vi "biref2.vi"() -> ()   [LabVIEW 2025]
doc: "Author: Scott Hannahs <sth@magnet.fsu.edu>\n\nThis software is licensed for use under the “MIT License\"\nCopyright (c) 2025 Scott Hannahs, sth@sth@magnet.sthnet.net\n\nPermission is hereby granted, free of charge, to any person obtaining a copy of this software and associated documentation files (the \"Software\"), to deal in the Software without restriction, including without limitation the rights to use, copy, modify, merge, publish, distribute, sublicense, and/or sell copies of the Software, and to permit persons to whom the Software is furnished to do so, subject to the following conditions: The above copyright notice and this permission notice shall be included in all copies or substantial portions of the Software.\n\nTHE SOFTWARE IS PROVIDED \"AS IS\", WITHOUT WARRANTY OF ANY KIND, EXPRESS OR IMPLIED, INCLUDING BUT NOT LIMITED TO THE WARRANTIES OF MERCHANTABILITY, FITNESS FOR A PARTICULAR PURPOSE AND NONINFRINGEMENT. IN NO EVENT SHALL THE AUTHORS OR COPYRIGHT HOLDERS BE LIABLE FOR ANY CLAIM, DAMAGES OR OTHER LIABILITY, WHETHER IN AN ACTION OF CONTRACT, TORT OR OTHERWISE, ARISING FROM, OUT OF OR IN CONNECTION WITH THE SOFTWARE OR THE USE OR OTHER DEALINGS IN THE SOFTWARE."
panel:
  in  "Case Constant\n(See Context Help)":bool
  in  "folder name":string
  in  "field increment":dbl
  out "Current field":dbl
  in  "Initial field T":dbl=0.08
  in  "No  Steps":i16
  out "outputdc 2":dbl[](array[numeric]) format="%.2f"
  in  "GPIB address dc meter 2":string="2"
  in  "GPIB address dc meter":string="5"
  in  "GPIB  address  lockin":string="3"
  in  "GPIB address magnet":string="1"
  in  "GPIB address Temp controller":string="12"
  in  "Wait (second)":sgl
  in  "No of Temp Steps":i16
  out "outputtemp":dbl[](array[numeric]) format="%.2f"
  out "outputdc":dbl[](array[numeric]) format="%.2f"
  out "outputlockin 2":dbl[](array[numeric]) format="%.2f"
  out "outputlockin 1":dbl[](array[numeric]) format="%.2f"
  out "field":dbl[](array[numeric]) format="%.2f"
  out "Current Temp":dbl format="%.3f"
  in  "Increasing \nTemp step":bool=TRUE
  in  "Initial Temp C":dbl format="%.3f"
  # "Help:\n1. write the folder name to save the files.The file name will \nbe the temperature in the given folder.\n2.Write the GPIB address of all the instruments before running\nthe program.\n3. Give the initial temperature and the temperature interval \nand the total number of steps.\n4.Check whether you want to increase the temperature or\ndecrease.\n5.Write the time to be waited to let the tempetature controller\nequilibrate.\n6.Once the speps 1 through 5 is done run the experiment."
  # "Decreasing\nTemp Step"
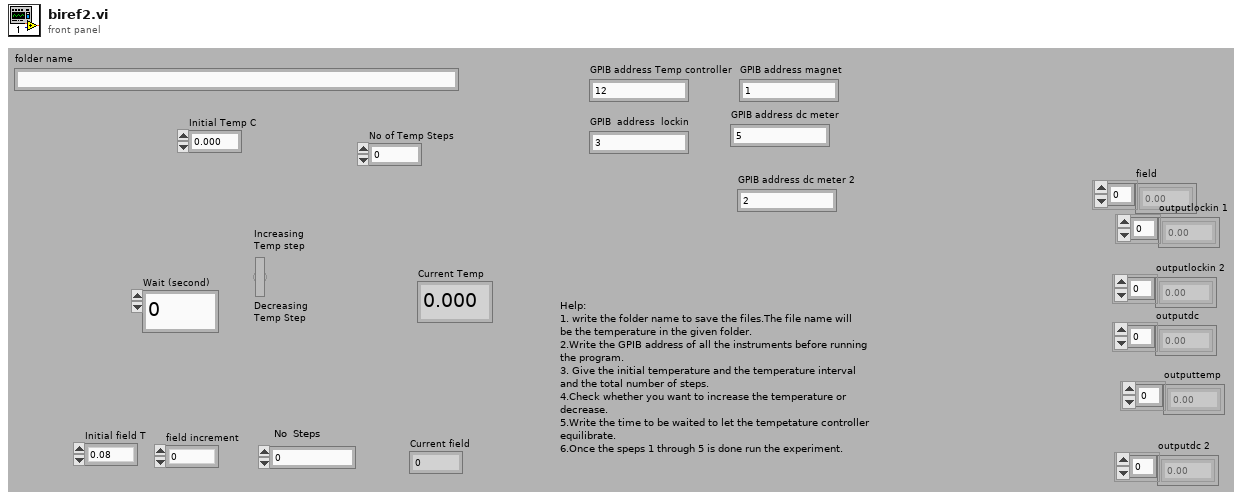
[diagram p1: front panel]
types:
  T1 = enum16{"--Quit--", "Read-Status", "Read-Cell", "Read-Field[T]", "Read-Setpoint[T]"}
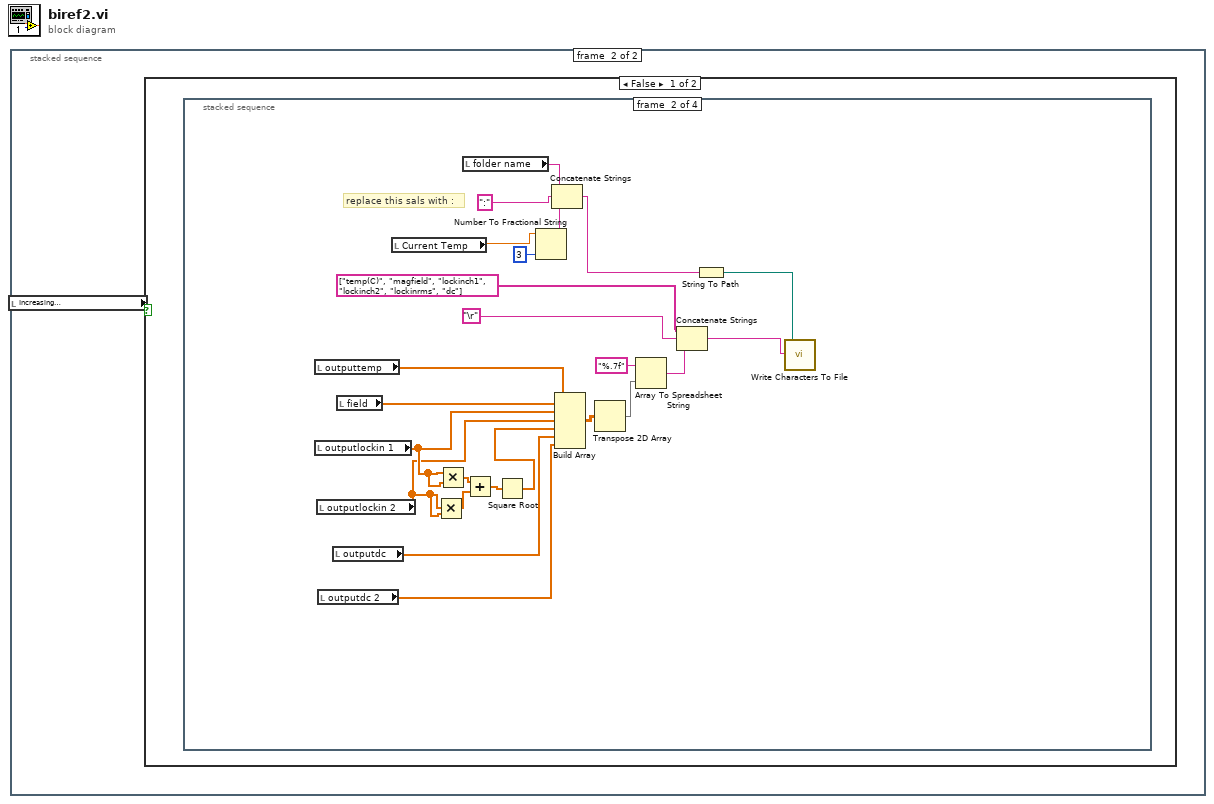
[diagram p0: block diagram]
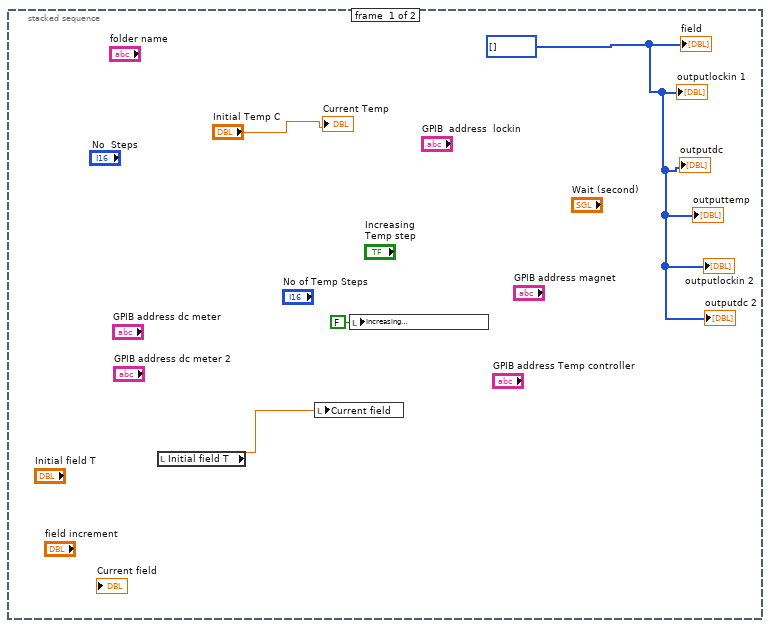
[diagram p2: hidden frame]
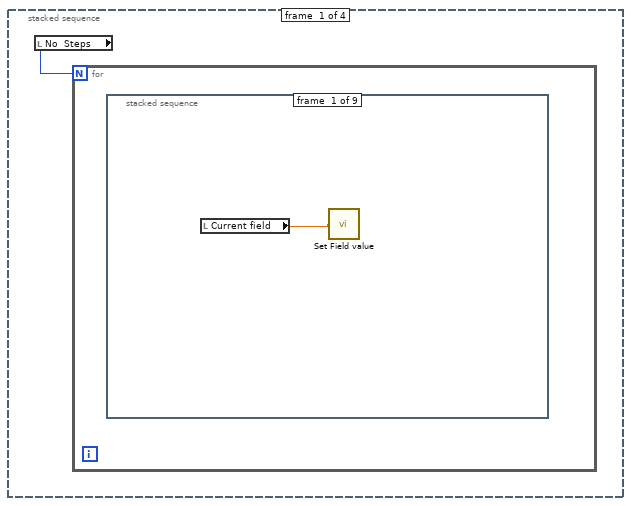
[diagram p3: hidden frame]
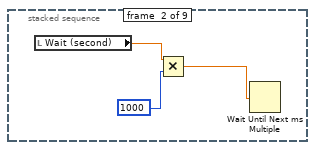
[diagram p4: hidden frame]
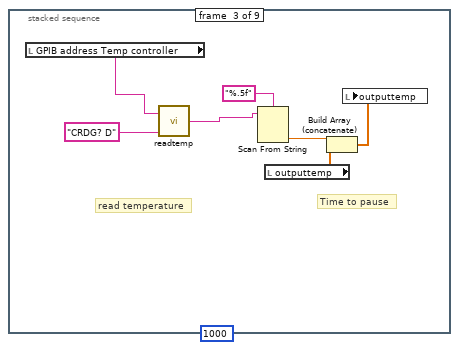
[diagram p5: hidden frame]
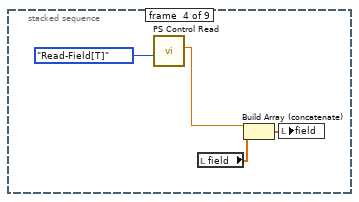
[diagram p6: hidden frame]
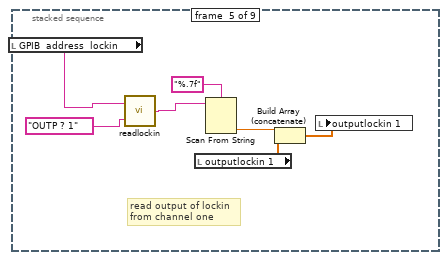
[diagram p7: hidden frame]
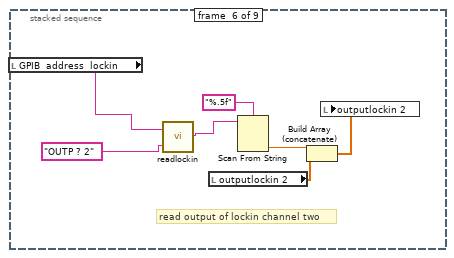
[diagram p8: hidden frame]
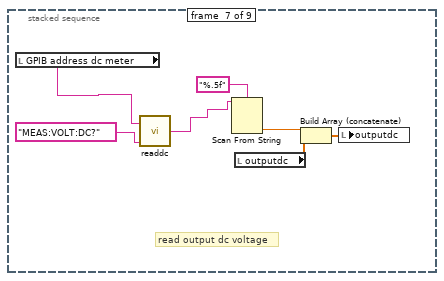
[diagram p9: hidden frame]
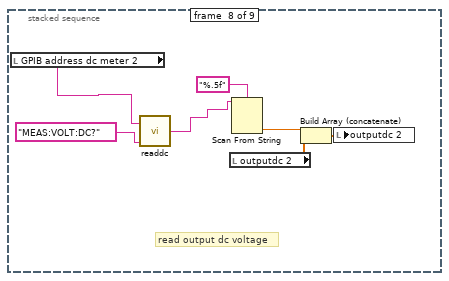
[diagram p10: hidden frame]
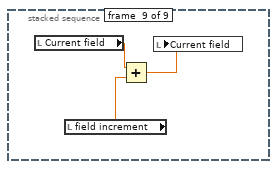
[diagram p11: hidden frame]
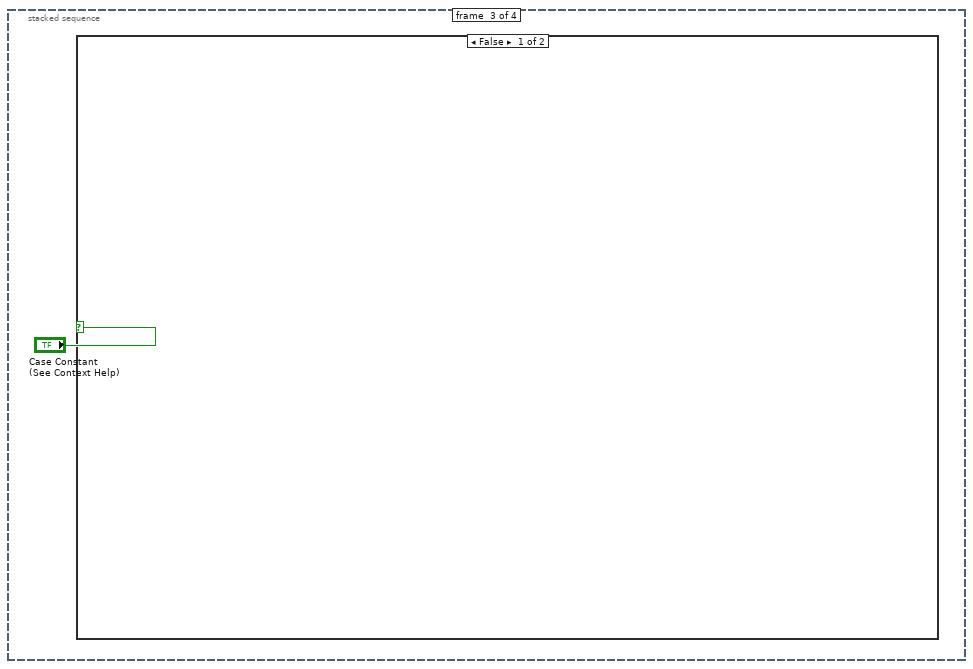
[diagram p12: hidden frame]
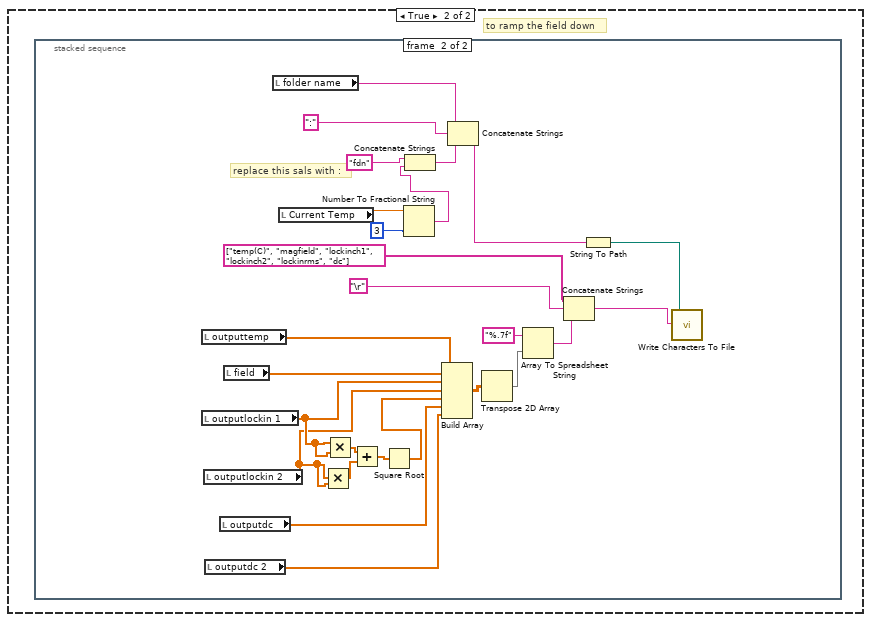
[diagram p13: hidden frame]
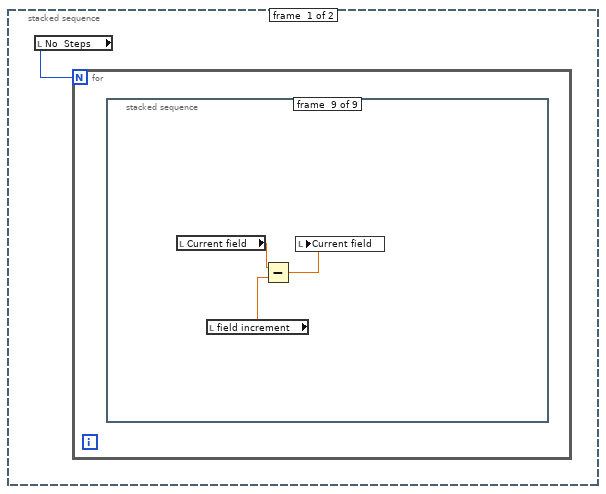
[diagram p14: hidden frame]
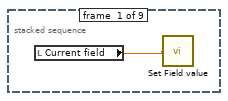
[diagram p15: hidden frame]
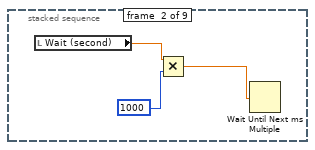
[diagram p16: hidden frame]
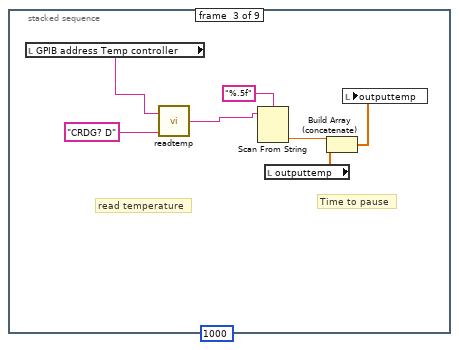
[diagram p17: hidden frame]
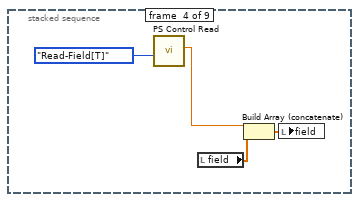
[diagram p18: hidden frame]
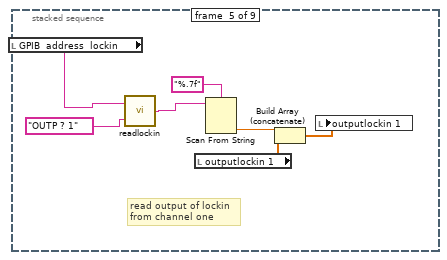
[diagram p19: hidden frame]
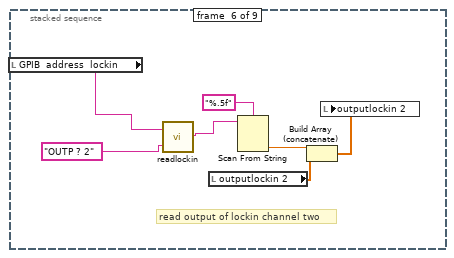
[diagram p20: hidden frame]
diagram:
  n1 = stacked-sequence {
    frame #0 {
      w3 = i32[] [] ("field")
      n2 = local read "Initial field T"() -> (w1:dbl)
      n3 = local write "Current field"(w1) -> ()
      n4 = local write "Increasing \nTemp step"(FALSE ("Increasing \nTemp step")) -> ()
      "Current Temp" <- "Initial Temp C"
      "field" <- w3
      "outputlockin 1" <- w3
      "outputdc" <- w3
      "outputtemp" <- w3
      "outputlockin 2" <- w3
      "outputdc 2" <- w3
    }
    frame #1 {
      n5 = local read "Increasing \nTemp step"() -> (w5:bool)
      n6 = case shown="False" w5 {
        frame False {
          n7 = stacked-sequence {
            frame #0 {
              n8 = local read "No  Steps"() -> (w6:i16)
              n9 = for {
                N: w6 -> [_]
                n10 = stacked-sequence {
                  frame #0 {
                    n11 = local read "Current field"() -> (w7:dbl)
                    n12 = call "Set Field value.vi"("Field"=w7) -> ()
                  }
                  frame #1 {
                    n13 = local read "Wait (second)"() -> (w10:sgl)
                    n14 = Multiply(x=w10, y=u32 1000 ("millisecond multiple")) -> (x*y=w8:sgl)
                    n15 = Wait Until Next ms Multiple(millisecond multiple=w8) -> ()  [unwired: 1 out]
                  }
                  frame #2 {
                    (unwired) u32 1000 ("millisecond multiple")
                    # "Time to pause"
                    # "read temperature"
                    n16 = local read "GPIB address Temp controller"() -> (w11:string)
                    n17 = call "readtemp.vi"("Characters to Write"="CRDG? D", "GPIB\nAddress"=w11) -> ("Characters Read"=w12:string)
                    n18 = Scan From String(format string="%.5f", input string=w12) -> (output 1=w14:dbl)  [unwired: 3 in, 3 out]
                    n19 = local read "outputtemp"() -> (w17:dbl[])
                    n20 = Build Array (concatenate)(w14, w17) -> (w16:dbl[])
                    n21 = local write "outputtemp"(w16) -> ()
                  }
                  frame #3 {
                    n22 = call "PS Control Read.vi"("Read State"=T1."Read-Field[T]") -> ("Current Field"=w18:dbl)  [unwired: 3 in, 4 out]
                    n23 = local read "field"() -> (w20:dbl[])
                    n24 = Build Array (concatenate)(w18, w20) -> (w19:dbl[])
                    n25 = local write "field"(w19) -> ()
                  }
                  frame #4 {
                    # "read output of lockin\nfrom channel one"
                    n26 = local read "GPIB  address  lockin"() -> (w22:string)
                    n27 = call "readlockin.vi"("Characters to Write"="OUTP ? 1", "GPIB\nAddress"=w22) -> ("Characters Read"=w23:string)
                    n28 = local read "outputlockin 1"() -> (w27:dbl[])
                    n29 = Scan From String(format string="%.7f", input string=w23) -> (output 1=w24:dbl)  [unwired: 3 in, 3 out]
                    n30 = Build Array (concatenate)(w24, w27) -> (w26:dbl[])
                    n31 = local write "outputlockin 1"(w26) -> ()
                  }
                  frame #5 {
                    # "read output of lockin channel two"
                    n32 = local read "GPIB  address  lockin"() -> (w29:string)
                    n33 = call "readlockin.vi"("Characters to Write"="OUTP ? 2", "GPIB\nAddress"=w29) -> ("Characters Read"=w30:string)
                    n34 = local read "outputlockin 2"() -> (w34:dbl[])
                    n35 = Scan From String(format string="%.5f", input string=w30) -> (output 1=w32:dbl)  [unwired: 3 in, 3 out]
                    n36 = Build Array (concatenate)(w32, w34) -> (w33:dbl[])
                    n37 = local write "outputlockin 2"(w33) -> ()
                  }
                  frame #6 {
                    # "read output dc voltage"
                    n38 = local read "GPIB address dc meter"() -> (w36:string)
                    n39 = call "readdc.vi"("Characters to Write"="MEAS:VOLT:DC?", "GPIB\nAddress"=w36) -> ("Characters Read"=w37:string)
                    n40 = Scan From String(format string="%.5f", input string=w37) -> (output 1=w39:dbl)  [unwired: 3 in, 3 out]
                    n41 = local read "outputdc"() -> (w42:dbl[])
                    n42 = Build Array (concatenate)(w39, w42) -> (w41:dbl[])
                    n43 = local write "outputdc"(w41) -> ()
                  }
                  frame #7 {
                    # "read output dc voltage"
                    n44 = local read "GPIB address dc meter 2"() -> (w43:string)
                    n45 = call "readdc.vi"("Characters to Write"="MEAS:VOLT:DC?", "GPIB\nAddress"=w43) -> ("Characters Read"=w44:string)
                    n46 = local read "outputdc 2"() -> (w49:dbl[])
                    n47 = Scan From String(format string="%.5f", input string=w44) -> (output 1=w46:dbl)  [unwired: 3 in, 3 out]
                    n48 = Build Array (concatenate)(w46, w49) -> (w48:dbl[])
                    n49 = local write "outputdc 2"(w48) -> ()
                  }
                  frame #8 {
                    n50 = local read "Current field"() -> (w52:dbl)
                    n51 = local read "field increment"() -> (w51:dbl)
                    n52 = Add(x=w52, y=w51) -> (x+y=w50:dbl)
                    n53 = local write "Current field"(w50) -> ()
                  }
                }
              }
            }
            frame #1 {
              # "replace this sals with :"
              n54 = local read "outputtemp"() -> (w71:dbl[])
              n55 = local read "outputlockin 1"() -> (w69:dbl[])
              n56 = local read "outputlockin 2"() -> (w68:dbl[])
              n57 = local read "outputdc 2"() -> (w54:dbl[])
              n58 = local read "outputdc"() -> (w63:dbl[])
              n59 = local read "field"() -> (w70:dbl[])
              n60 = local read "Current Temp"() -> (w73:dbl)
              n61 = Multiply(x=w68, y=w68) -> (x*y=w66:dbl[])
              n62 = Multiply(x=w69, y=w69) -> (x*y=w67:dbl[])
              n63 = local read "folder name"() -> (w53:string)
              n64 = Add(x=w67, y=w66) -> (x+y=w65:dbl[])
              n65 = Square Root(x=w65) -> (sqrt(x)=w64:dbl[])
              n66 = Number To Fractional String(number=w73, precision (6)=i16 3) -> (F-format string=w72:string)  [unwired: 2 in]
              n67 = Concatenate Strings(w53, ":", w72) -> (w75:string)
              n68 = Build Array(w71, w70, w69, w68, w64, w63, w54) -> (w62:dbl[][])
              n69 = Transpose 2D Array(2D array=w62) -> (transposed array=w60:dbl[][])
              n70 = Array To Spreadsheet String(array=w60, 3:"%.7f" ("format string")) -> (spreadsheet string=w57:string)  [unwired: 1 in]
              n71 = Concatenate Strings(string[] ["temp(C)", "magfield", "lockinch1", "lockinch2", "lockinrms", "dc"], "\r", w57) -> (w56:string)
              n72 = String To Path(string=w75) -> (path=w74:path)
              n73 = call <vilib>:"Write Characters To File.vi"("character string"=w56, "file path (dialog if empty)"=w74) -> ()  [unwired: 3 in, 1 out]
            }
            frame #2 {
              n74 = case shown="False" "Case Constant\n(See Context Help)" {
                frame False {
                }
                frame True {
                  # "to ramp the field down"
                  n75 = stacked-sequence {
                    frame #0 {
                      n76 = local read "No  Steps"() -> (w78:i16)
                      n77 = for {
                        N: w78 -> [_]
                        n78 = stacked-sequence {
                          frame #0 {
                            n79 = local read "Current field"() -> (w79:dbl)
                            n80 = call "Set Field value.vi"("Field"=w79) -> ()
                          }
                          frame #1 {
                            n81 = local read "Wait (second)"() -> (w82:sgl)
                            n82 = Multiply(x=w82, y=u32 1000 ("millisecond multiple")) -> (x*y=w80:sgl)
                            n83 = Wait Until Next ms Multiple(millisecond multiple=w80) -> ()  [unwired: 1 out]
                          }
                          frame #2 {
                            (unwired) u32 1000 ("millisecond multiple")
                            # "Time to pause"
                            # "read temperature"
                            n84 = local read "GPIB address Temp controller"() -> (w83:string)
                            n85 = call "readtemp.vi"("Characters to Write"="CRDG? D", "GPIB\nAddress"=w83) -> ("Characters Read"=w84:string)
                            n86 = Scan From String(format string="%.5f", input string=w84) -> (output 1=w86:dbl)  [unwired: 3 in, 3 out]
                            n87 = local read "outputtemp"() -> (w89:dbl[])
                            n88 = Build Array (concatenate)(w86, w89) -> (w88:dbl[])
                            n89 = local write "outputtemp"(w88) -> ()
                          }
                          frame #3 {
                            n90 = call "PS Control Read.vi"("Read State"=T1."Read-Field[T]") -> ("Current Field"=w90:dbl)  [unwired: 3 in, 4 out]
                            n91 = local read "field"() -> (w92:dbl[])
                            n92 = Build Array (concatenate)(w90, w92) -> (w91:dbl[])
                            n93 = local write "field"(w91) -> ()
                          }
                          frame #4 {
                            # "read output of lockin\nfrom channel one"
                            n94 = local read "GPIB  address  lockin"() -> (w94:string)
                            n95 = call "readlockin.vi"("Characters to Write"="OUTP ? 1", "GPIB\nAddress"=w94) -> ("Characters Read"=w95:string)
                            n96 = local read "outputlockin 1"() -> (w99:dbl[])
                            n97 = Scan From String(format string="%.7f", input string=w95) -> (output 1=w96:dbl)  [unwired: 3 in, 3 out]
                            n98 = Build Array (concatenate)(w96, w99) -> (w98:dbl[])
                            n99 = local write "outputlockin 1"(w98) -> ()
                          }
                          frame #5 {
                            # "read output of lockin channel two"
                            n100 = local read "GPIB  address  lockin"() -> (w101:string)
                            n101 = call "readlockin.vi"("Characters to Write"="OUTP ? 2", "GPIB\nAddress"=w101) -> ("Characters Read"=w102:string)
                            n102 = local read "outputlockin 2"() -> (w106:dbl[])
                            n103 = Scan From String(format string="%.5f", input string=w102) -> (output 1=w104:dbl)  [unwired: 3 in, 3 out]
                            n104 = Build Array (concatenate)(w104, w106) -> (w105:dbl[])
                            n105 = local write "outputlockin 2"(w105) -> ()
                          }
                          frame #6 {
                            # "read output dc voltage"
                            n106 = local read "GPIB address dc meter"() -> (w108:string)
                            n107 = call "readdc.vi"("Characters to Write"="MEAS:VOLT:DC?", "GPIB\nAddress"=w108) -> ("Characters Read"=w109:string)
                            n108 = Scan From String(format string="%.5f", input string=w109) -> (output 1=w111:dbl)  [unwired: 3 in, 3 out]
                            n109 = local read "outputdc"() -> (w114:dbl[])
                            n110 = Build Array (concatenate)(w111, w114) -> (w113:dbl[])
                            n111 = local write "outputdc"(w113) -> ()
                          }
                          frame #7 {
                            # "read output dc voltage"
                            n112 = local read "GPIB address dc meter 2"() -> (w115:string)
                            n113 = call "readdc.vi"("Characters to Write"="MEAS:VOLT:DC?", "GPIB\nAddress"=w115) -> ("Characters Read"=w116:string)
                            n114 = local read "outputdc 2"() -> (w121:dbl[])
                            n115 = Scan From String(format string="%.5f", input string=w116) -> (output 1=w118:dbl)  [unwired: 3 in, 3 out]
                            n116 = Build Array (concatenate)(w118, w121) -> (w120:dbl[])
                            n117 = local write "outputdc 2"(w120) -> ()
                          }
                          frame #8 {
                            n118 = local read "Current field"() -> (w124:dbl)
                            n119 = local read "field increment"() -> (w123:dbl)
                            n120 = Subtract(x=w124, y=w123) -> (x-y=w122:dbl)
                            n121 = local write "Current field"(w122) -> ()
                          }
                        }
                      }
                    }
                    frame #1 {
                      # "replace this sals with :"
                      n122 = local read "outputtemp"() -> (w146:dbl[])
                      n123 = local read "outputlockin 1"() -> (w144:dbl[])
                      n124 = local read "outputlockin 2"() -> (w143:dbl[])
                      n125 = local read "outputdc 2"() -> (w129:dbl[])
                      n126 = local read "outputdc"() -> (w138:dbl[])
                      n127 = local read "field"() -> (w145:dbl[])
                      n128 = local read "folder name"() -> (w128:string)
                      n129 = local read "Current Temp"() -> (w147:dbl)
                      n130 = Multiply(x=w143, y=w143) -> (x*y=w141:dbl[])
                      n131 = Multiply(x=w144, y=w144) -> (x*y=w142:dbl[])
                      n132 = Add(x=w142, y=w141) -> (x+y=w140:dbl[])
                      n133 = Square Root(x=w140) -> (sqrt(x)=w139:dbl[])
                      n134 = Number To Fractional String(number=w147, precision (6)=i16 3) -> (F-format string=w127:string)  [unwired: 2 in]
                      n135 = Concatenate Strings("fdn", w127) -> (w125:string)
                      n136 = Build Array(w146, w145, w144, w143, w139, w138, w129) -> (w137:dbl[][])
                      n137 = Concatenate Strings(w128, ":", w125) -> (w149:string)
                      n138 = Transpose 2D Array(2D array=w137) -> (transposed array=w135:dbl[][])
                      n139 = Array To Spreadsheet String(array=w135, 3:"%.7f" ("format string")) -> (spreadsheet string=w132:string)  [unwired: 1 in]
                      n140 = Concatenate Strings(string[] ["temp(C)", "magfield", "lockinch1", "lockinch2", "lockinrms", "dc"], "\r", w132) -> (w131:string)
                      n141 = String To Path(string=w149) -> (path=w148:path)
                      n142 = call <vilib>:"Write Characters To File.vi"("character string"=w131, "file path (dialog if empty)"=w148) -> ()  [unwired: 3 in, 1 out]
                    }
                  }
                }
              }
            }
            frame #3 {
              w151 = i32[] []
              n143 = local write "outputlockin 2"(w151) -> ()
              n144 = local write "outputtemp"(w151) -> ()
              n145 = local write "outputlockin 1"(w151) -> ()
              n146 = local write "outputdc"(w151) -> ()
              n147 = local write "field"(w151) -> ()
            }
          }
        }
        frame True {
          n148 = local read "No of Temp Steps"() -> (w152:i16)
          n149 = for {
            N: w152 -> [_]
          }
        }
      }
    }
  }
